vi "SkipMusic.vi"(0 "reference in":refnum<class "MediaPlayer.lvclass">, 11 "Error In":errorcluster) -> (4 "reference out":refnum<class "MediaPlayer.lvclass">, 15 "Error Out":errorcluster)   [LabVIEW 2024, in "MediaPlayer.lvclass"]
doc: "Skips current music and pauses it."
uses:
  MediaPlayer.lvclass
panel:
  # "Connector Pane"
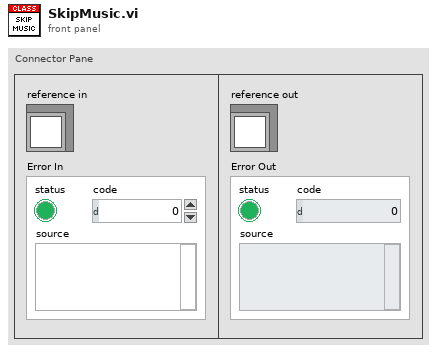
[diagram p1: front panel]
types:
  T1 = typedef "MediaPlayer.lvclass/ObjectAttributes.ctl" = cluster{"MediaPlayerData":T2, "Current Info":T4}
  T2 = typedef "MediaPlayer.lvclass/MediaPlayer Data.ctl" = cluster{"Music List":path[], "Current Music Index":i64, "Song Handler":T3, "Device ID":u32}
  T3 = typedef "Sound Output Task ID.ctl" = u32
  T4 = typedef "MediaPlayer.lvclass/Current Info.ctl" = cluster{"Duration":dbl, "Name":string, "Is playing?":bool, "Current Music Index":i64}
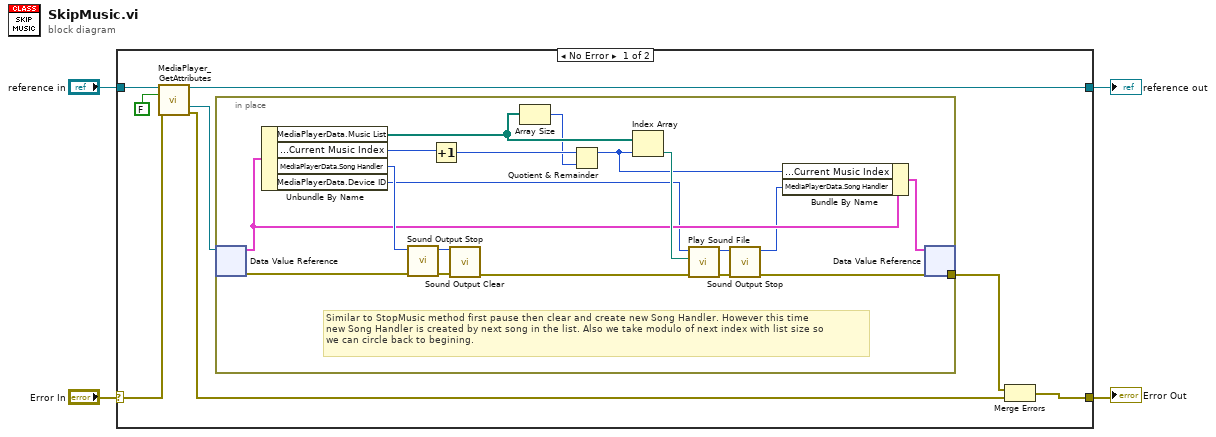
[diagram p0: block diagram]
diagram:
  n1 = case shown="No Error" "Error In" {
    selector: "Error In" -> [w11 w32]
    tunnel: [w6 w32] -> w3
    tunnel: [w10 w31] -> w1
    tunnel: "reference in" -> [w12 w31]
    frame No Error {
      n2 = call "MediaPlayer_GetAttributes.vi"("reference in"=w12, "OnlyGetDvrReference(False)"=FALSE, "Error In"=w11) -> ("reference out"=w10:refnum<class "MediaPlayer.lvclass">, "DataRef"=w7:refnum<data-value>, "Error Out"=w8:errorcluster)  [unwired: 9 in, 1 out]
      n3 = in-place {
        in-place-border: [w19] -> w5
        # "Similar to StopMusic method first pause then clear and create new Song Handler. However this time\nnew Song Handler is created by next song in the list. Also we take modulo of next index with list size so\nwe can circle back to begining."
        n4 = in-place-dvr #1(w7) -> (w23:T1, w25:errorcluster)
        n5 = Unbundle By Name(w23) -> ("MediaPlayerData.Music List"=w16:path[], "MediaPlayerData.Current Music Index"=w30:i64, "MediaPlayerData.Song Handler"=w26:T3, "MediaPlayerData.Device ID"=w20:u32)
        n6 = call <vilib>:"Sound Output Stop.vi"("error in (no error)"=w25, "task ID"=w26) -> ("error out"=w29:errorcluster, "task ID out"=w28:T3)  [unwired: 8 in]
        n7 = Increment(x=w30) -> (x+1=w15:i64)
        n8 = call <vilib>:"Sound Output Clear.vi"("error in (no error)"=w29, "task ID"=w28) -> ("error out"=w27:errorcluster)  [unwired: 9 in]
        n9 = Array Size(array=w16) -> (size(s)=w14:i32)
        n10 = Quotient & Remainder(x=w15, y=w14) -> (x-y*floor(x/y)=w13:i64)  [unwired: 1 out]
        n11 = Index Array(array=w16, index=w13) -> (element=w24:path)
        n12 = call <vilib>:"Play Sound File.vi"("error in (no error)"=w27, "path"=w24, "device ID"=w20) -> ("error out"=w21:errorcluster, "task ID"=w18:T3)  [unwired: 7 in]
        n13 = call <vilib>:"Sound Output Stop.vi"("error in (no error)"=w21, "task ID"=w18) -> ("error out"=w19:errorcluster, "task ID out"=w17:T3)  [unwired: 8 in]
        n14 = Bundle By Name(cluster=w23, "MediaPlayerData.Current Music Index"=w13, "MediaPlayerData.Song Handler"=w17) -> (w22:T1)
        n15 = in-place-dvr #1(w22) -> ()  [unwired: 2 out]
      }
      n16 = Merge Errors(w5, w8) -> (w6:errorcluster)
    }
    frame Error {
    }
  }
  "Error Out" <- w3
  "reference out" <- w1
